vi "ReadRestart.vi"(8 "error in (no error)":errorcluster, 11 "object in":refnum<class "shutdown_reply Message.lvclass">) -> (0 "error out":errorcluster, 2 "restart":bool, 3 "object out":refnum<class "shutdown_reply Message.lvclass">)   [LabVIEW 2018, in "ClientMessaging.lvlib" / "shutdown_reply Message.lvclass"]
uses:
  shutdown_reply Message.lvclass
  shutdown_reply Message.lvclass/shutdown_reply Message.ctl
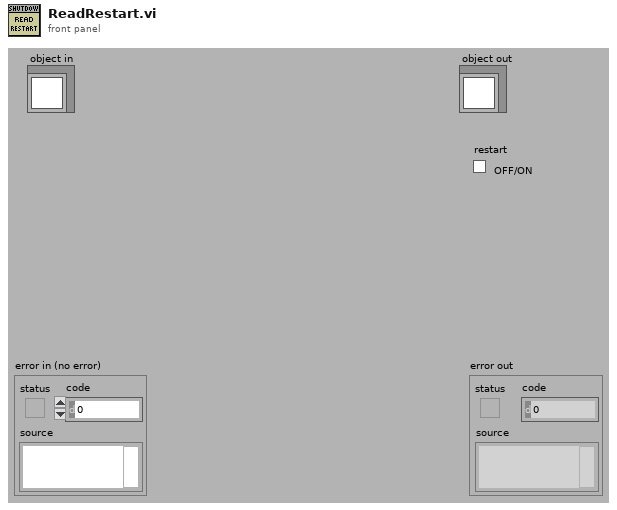
[diagram p1: front panel]
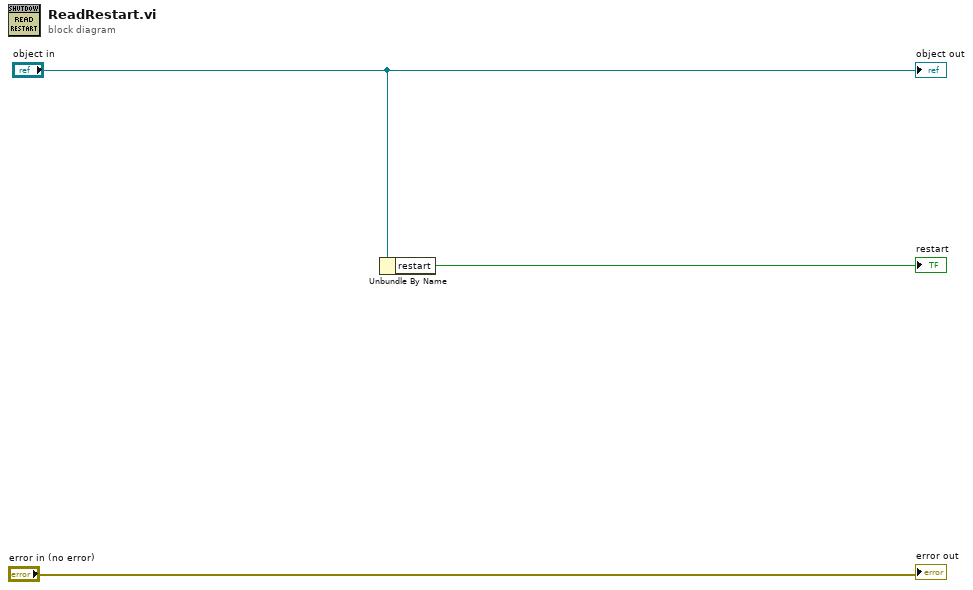
[diagram p0: block diagram]
diagram:
  n1 = Unbundle By Name("object in") -> ("restart"=→"restart":bool)
  "error out" <- "error in (no error)"
  "object out" <- "object in"
